vi "Get Cluster Element by Name__ogtk.vi"(8 "error in (no error)":errorcluster, 9 "Element Name":string, 10 "Cluster":variant) -> (0 "error out":errorcluster, 1 "found?":bool, 2 "VElement":variant)   [LabVIEW 2016]
doc: "Returns the element in the cluster by its name."
panel:
  # "[OpenG VI Tags] ***Do Not Remove***"
  # "Get Cluster Element by Name.vi\n\nReturns the element in the cluster by its name.\n\nPlease visit http://www.OpenG.org to learn about the\nOpen Source LabVIEW software movement.\n\nNOTICE -- YOU MUST LEAVE THIS NOTICE IN PLACE.  PER THE TERMS OF THE LICENSE BELOW, YOU MAY SUBLICENSE THIS SOFTWARE \nIN ANY WAY THAT DOES NOT CONFLICT WITH THIS LICENSE.\n\n### BSD License (http://www.opensource.org/licenses/bsd-license.php) Begin ###\n \nCopyright (c) 2002, Jean-Pierre Drolet <drolet_jp@hotmail.com>\nCopyright (c) 2002-2006, Jim Kring <jim@jimkring.com>\n\nAll rights reserved.\n\nRedistribution and use in source and binary forms, with or without modification, are permitted provided that the following conditions are met:\n\n    * Redistributions of source code must retain the above copyright notice, this list of conditions and the following disclaimer.\n    * Redistributions in binary form must reproduce the above copyright notice, this list of conditions and the following disclaimer in the \n       documentation and/or other materials provided with the distribution.\n    * Neither the name of SciWare, James Kring, Inc., nor the names of its contributors may be used to endorse or promote products derived \n       from this software without specific prior written permission.\n\nTHIS SOFTWARE IS PROVIDED BY THE COPYRIGHT HOLDERS AND CONTRIBUTORS \"AS IS\" AND ANY EXPRESS OR IMPLIED WARRANTIES, \nINCLUDING, BUT NOT LIMITED TO, THE IMPLIED WARRANTIES OF MERCHANTABILITY AND FITNESS FOR A PARTICULAR PURPOSE ARE \nDISCLAIMED. IN NO EVENT SHALL THE COPYRIGHT OWNER OR CONTRIBUTORS BE LIABLE FOR ANY DIRECT, INDIRECT, INCIDENTAL,\n SPECIAL, EXEMPLARY, OR CONSEQUENTIAL DAMAGES (INCLUDING, BUT NOT LIMITED TO, PROCUREMENT OF SUBSTITUTE GOODS OR \nSERVICES; LOSS OF USE, DATA, OR PROFITS; OR BUSINESS INTERRUPTION) HOWEVER CAUSED AND ON ANY THEORY OF LIABILITY, \nWHETHER IN CONTRACT, STRICT LIABILITY, OR TORT (INCLUDING NEGLIGENCE OR OTHERWISE) ARISING IN ANY WAY OUT OF THE USE \nOF THIS SOFTWARE, EVEN IF ADVISED OF THE POSSIBILITY OF SUCH DAMAGE.\n\n### BSD License End ###\nFoundation, Inc., 59 Temple Place, Suite 330, Boston, MA 02111-1307 USA"
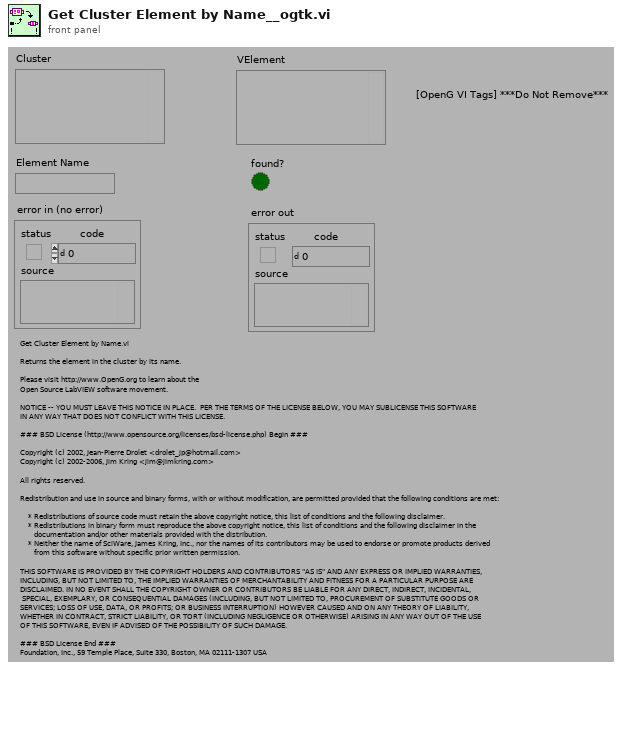
[diagram p1: front panel]
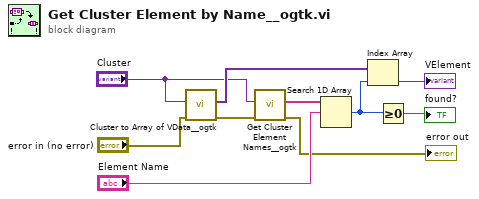
[diagram p0: block diagram]
diagram:
  n1 = call <userlib>:"Cluster to Array of VData__ogtk.vi"("error in (no error)"="error in (no error)", "Cluster"="Cluster") -> ("error out"=w4:errorcluster, "Array of VData"=w9:variant[])  [unwired: 8 in]
  n2 = call <userlib>:"Get Cluster Element Names__ogtk.vi"("error in (no error)"=w4, "Cluster"="Cluster") -> ("error out"=→"error out":errorcluster, "Element Names"=w3:string[])  [unwired: 8 in]
  n3 = Search 1D Array(1D array=w3, element="Element Name") -> (index of element=w7:i32)  [unwired: 1 in]
  n4 = Index Array(array=w9, index=w7) -> (element=→"VElement":variant)
  n5 = Greater Or Equal To 0?(x=w7) -> (x >= 0?=→"found?":bool)
